vi "Teleop - Elevator Control.vi"(9 "Joystick 0 Axes":dbl[](array[numeric]), 10 "Buttons":bool[](array[boolean]), 11 "Joystick 1 Axes":dbl[](array[numeric])) -> ()   [LabVIEW 2017]
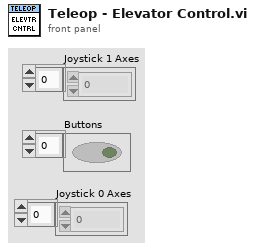
[diagram p1: front panel]
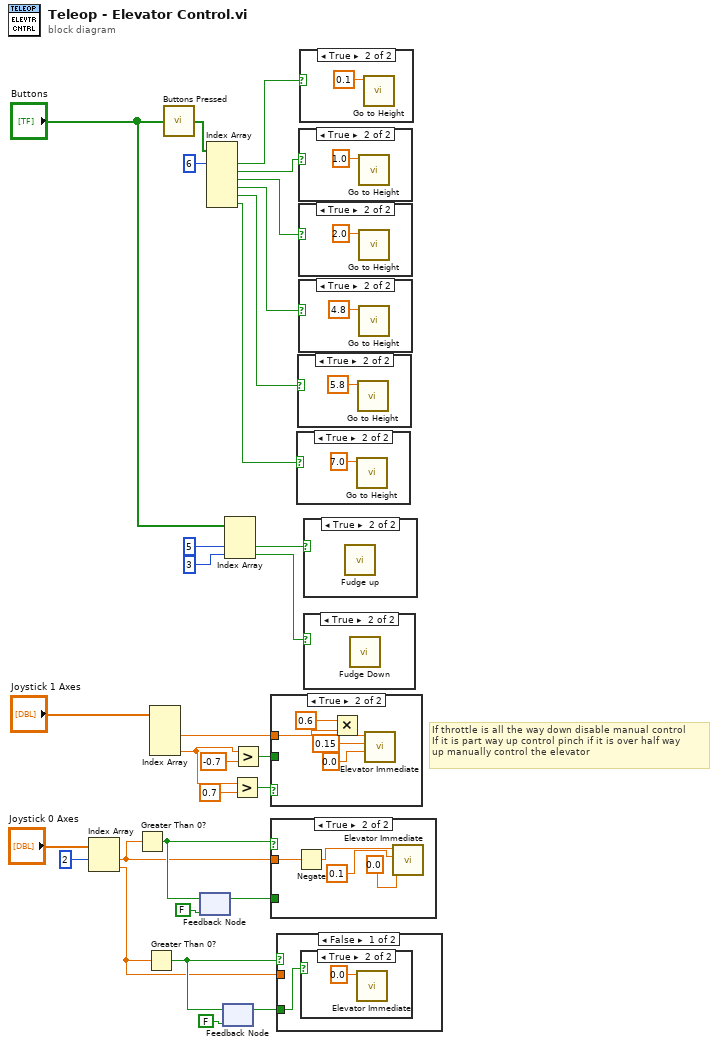
[diagram p0: block diagram]
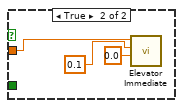
[diagram p3: hidden frame]
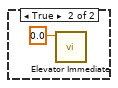
[diagram p5: hidden frame]
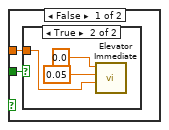
[diagram p10: hidden frame]
diagram:
  # "If throttle is all the way down disable manual control\nIf it is part way up control pinch if it is over half way\nup manually control the elevator"
  n1 = Index Array(array="Joystick 0 Axes", index #1=2 ("index")) -> (element #1=w3:dbl, element #2=w2:dbl)  [unwired: 1 in]
  n2 = Greater Than 0?(x=w3) -> (x > 0?=w5:bool)
  n3 = Greater Than 0?(x=w2) -> (x > 0?=w6:bool)
  n4 = Index Array(array="Joystick 1 Axes") -> (element #2=w19:dbl, element #4=w24:dbl)  [unwired: 4 in, 2 out]
  n5 = call "Buttons Pressed.vi"("Button Values"="Buttons") -> ("Button Presses"=w11:bool[])
  n6 = feedback #1(FALSE) -> (w8:bool)
  n7 = feedback-in #1(w5) -> ()
  n8 = Index Array(array=w11, index #1=6 ("index")) -> (element #1=w12:bool, element #2=w13:bool, element #3=w25:bool, element #4=w26:bool, element #5=w27:bool, element #6=w28:bool)  [unwired: 5 in]
  n9 = feedback #2(FALSE) -> (w7:bool)
  n10 = feedback-in #2(w6) -> ()
  n11 = Index Array(array="Buttons", index #2=5 ("index"), index #3=3 ("index")) -> (element #2=w14:bool, element #3=w15:bool)  [unwired: 1 in, 1 out]
  n12 = Greater?(x=w24, y=0.7) -> (0:w21:bool)
  n13 = Greater?(x=w24, y=-0.7) -> (0:w23:bool)
  n14 = case shown="True" w21 {
    tunnel: w19 -> [w31 w40]
    tunnel: w23 -> [w32 _]
    frame False {
      n15 = case shown="True" w32 {
        tunnel: w31 -> [_ w33]
        frame False {
        }
        frame True {
          n16 = call "Elevator Immediate.vi"("Setpoint Pinch"=w33, "Deadband Value"=0.05, "Setpoint"=0.0 ("Setpoint Pinch")) -> ()  [unwired: 8 in, 1 out]
        }
      }
    }
    frame True {
      n17 = Multiply(x=0.6 ("y"), y=w40) -> (x*y=w37:dbl)
      n18 = call "Elevator Immediate.vi"("Setpoint Pinch"=0.0, "Deadband Value"=0.15, "Setpoint"=w37) -> ()  [unwired: 8 in, 1 out]
    }
  }
  n19 = case shown="True" w5 {
    tunnel: w3 -> [_ w46]
    tunnel: w8 -> [w41 _]
    frame False {
      n20 = case shown="False" w41 {
        frame False {
        }
        frame True {
          n21 = call "Elevator Immediate.vi"("Setpoint"=0.0) -> ()  [unwired: 10 in, 1 out]
        }
      }
    }
    frame True {
      n22 = Negate(x=w46) -> (-x=w45:dbl)
      n23 = call "Elevator Immediate.vi"("Setpoint Pinch"=0.0, "Deadband Value"=0.1, "Setpoint"=w45) -> ()  [unwired: 8 in, 1 out]
    }
  }
  n24 = case shown="False" w6 {
    tunnel: w2 -> [_ w51]
    tunnel: w7 -> [w47 _]
    frame False {
      n25 = case shown="True" w47 {
        frame False {
        }
        frame True {
          n26 = call "Elevator Immediate.vi"("Setpoint"=0.0) -> ()  [unwired: 10 in, 1 out]
        }
      }
    }
    frame True {
      n27 = call "Elevator Immediate.vi"("Setpoint Pinch"=0.0, "Deadband Value"=0.1, "Setpoint"=w51) -> ()  [unwired: 8 in, 1 out]
    }
  }
  n28 = case shown="True" w28 {
    frame False {
    }
    frame True {
      n29 = call "Go to Height.vi"("Target Height (in)"=7.0 ("Setpoint")) -> ()  [unwired: 10 in, 1 out]
    }
  }
  n30 = case shown="True" w27 {
    frame False {
    }
    frame True {
      n31 = call "Go to Height.vi"("Target Height (in)"=5.8 ("Setpoint")) -> ()  [unwired: 10 in, 1 out]
    }
  }
  n32 = case shown="True" w13 {
    frame False {
    }
    frame True {
      n33 = call "Go to Height.vi"("Target Height (in)"=1.0 ("Setpoint")) -> ()  [unwired: 10 in, 1 out]
    }
  }
  n34 = case shown="True" w25 {
    frame False {
    }
    frame True {
      n35 = call "Go to Height.vi"("Target Height (in)"=2.0 ("Setpoint")) -> ()  [unwired: 10 in, 1 out]
    }
  }
  n36 = case shown="True" w26 {
    frame False {
    }
    frame True {
      n37 = call "Go to Height.vi"("Target Height (in)"=4.8 ("Setpoint")) -> ()  [unwired: 10 in, 1 out]
    }
  }
  n38 = case shown="True" w12 {
    frame False {
    }
    frame True {
      n39 = call "Go to Height.vi"("Target Height (in)"=0.1 ("Setpoint")) -> ()  [unwired: 10 in, 1 out]
    }
  }
  n40 = case shown="True" w14 {
    frame False {
    }
    frame True {
      n41 = call "Fudge up.vi"() -> ()  [unwired: 11 in, 1 out]
    }
  }
  n42 = case shown="True" w15 {
    frame False {
    }
    frame True {
      n43 = call "Fudge Down.vi"() -> ()  [unwired: 11 in, 1 out]
    }
  }
